vi "ExSubSetupCam.vi"(2 "error in (no error)":errorcluster, 3 "Camera Handle":u32) -> (0 "error out":errorcluster, 1 "Camera Handle":u32)   [LabVIEW 2010]
panel:
  # "ExSubSetupCam:\nThis Sub VI sets up the skips, cleans, and shutter parameters.\nThis should be changed to suit the camera being used"
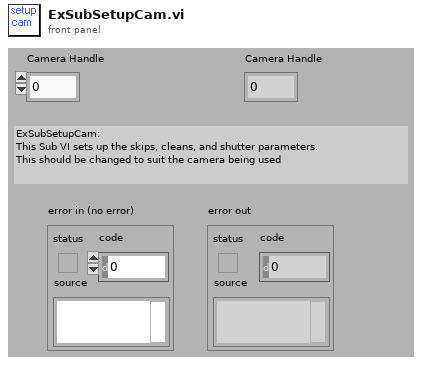
[diagram p1: front panel]
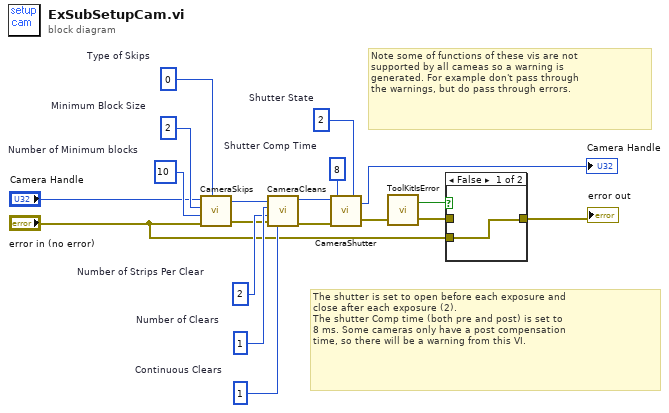
[diagram p0: block diagram]
diagram:
  w10 = u32 0  # Type of Skips
  w11 = u32 2  # Minimum Block Size
  w9 = u32 10  # Number of Minimum blocks
  w13 = u32 1  # Number of Clears
  w12 = u32 2  # Number of Strips Per Clear
  w14 = u32 1  # Continuous Clears
  w15 = u32 2  # Shutter State
  w16 = u32 8  # Shutter Comp Time
  # "Note some of functions of these vis are not \nsupported by all cameas so a warning is \ngenerated. For example don't pass through \nthe warnings, but do pass through errors."
  # "The shutter is set to open before each exposure and\nclose after each exposure (2).\nThe shutter Comp time (both pre and post) is set to \n8 ms. Some cameras only have a post compensation \ntime, so there will be a warning from this VI."
  n1 = call <userlib>:"CameraSkips.vi"("Camera Handle"="Camera Handle", "Minimum Block Size"=w11, "Number of Minimum blocks"=w9, "error in"="error in (no error)", "Type of Skips"=w10) -> ("Camera Handle"=w8:u32, "error out"=w7:errorcluster)
  n2 = call <userlib>:"CameraCleans.vi"("Camera Handle"=w8, "Number of Clears"=w13, "Number of Strips Per Clear"=w12, "error in"=w7, "Continuous Clears"=w14) -> ("Camera Handle"=w17:u32, "error out"=w18:errorcluster)
  n3 = call <userlib>:"CameraShutter.vi"("Camera Handle"=w17, "Shutter Comp Time: Pre Open"=w16, "Shutter Comp Time: Post Open"=w16, "error in"=w18, "Shutter State"=w15) -> ("Camera Handle"=→"Camera Handle":u32, "error out"=w5:errorcluster)
  n4 = call <userlib>:"ToolKitIsError.vi"("error in"=w5) -> ("error out"=w3:errorcluster, "Error Flag"=w4:bool)  [unwired: 1 in]
  n5 = case shown="False" w4 {
    tunnel: w3 -> [_ w21]
    tunnel: [w20 w21] -> w2
    tunnel: "error in (no error)" -> [w20 _]
    frame False {
    }
    frame True {
    }
  }
  "error out" <- w2
